vi "Configure Sweep Table.vi"(7 "Source Axis (1: swpOuter)":i32(ring)=1 items=["swpInner", "swpOuter"], 8 "error in (no error)":errorcluster, 9 "Table Column Index (0)":i32, 10 "Table File Name (\"MyFile.txt\")":string="\"MyFile.txt\"", 11 "VISA resource name":refnum<visa-resource-name>) -> (0 "error out":errorcluster, 3 "VISA resource name out":refnum<visa-resource-name>)   [LabVIEW 2014, in "Stanford Research SR1.lvlib"]
doc: "Sets the table filename used in conjunction with table-driven internalsweeps. The\ndefault directory for table sweep files is the \"user\" directory. Thus, filenames\nspecified without any additional path information will be expected to be found in\nthe \"user\" directory."
uses:
  Stanford Research SR1.lvlib
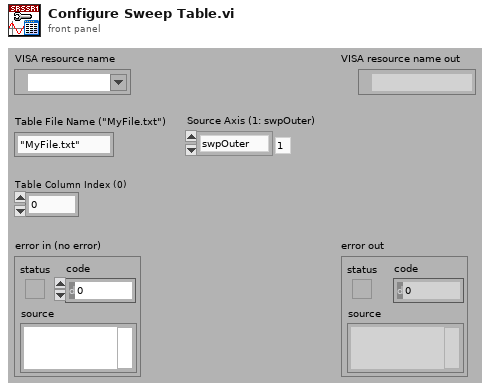
[diagram p1: front panel]
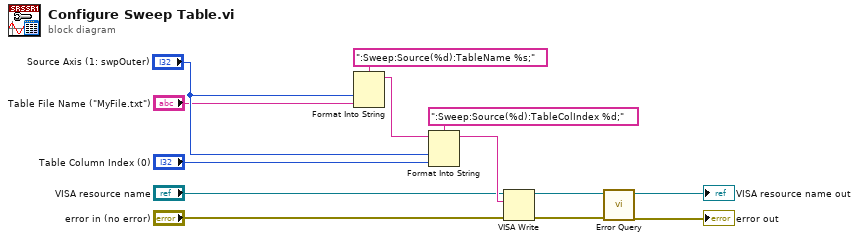
[diagram p0: block diagram]
diagram:
  n1 = Format Into String(format string=":Sweep:Source(%d):TableName %s;", "Source Axis (1: swpOuter)", "Table File Name (\"MyFile.txt\")") -> (resulting string=w12:string)  [unwired: 2 in, 1 out]
  n2 = Format Into String(format string=":Sweep:Source(%d):TableColIndex %d;", initial string=w12, "Source Axis (1: swpOuter)", "Table Column Index (0)") -> (resulting string=w10:string)  [unwired: 1 in, 1 out]
  n3 = VISA Write(VISA resource name="VISA resource name", write buffer=w10, error in (no error)="error in (no error)") -> (VISA resource name out=w7:refnum<visa-resource-name>, error out=w6:errorcluster)  [unwired: 1 out]
  n4 = call "Error Query.vi"("error in (no error)"=w6, "VISA resource name"=w7) -> ("error out"=→"error out":errorcluster, "VISA resource name out"=→"VISA resource name out":refnum<visa-resource-name>)  [unwired: 6 in, 2 out]
